vi "Get - SigMath Data.vi"(0 "reference in":refnum<class "SigMath.lvclass">, 5 "error in (no error)":errorcluster) -> (13 "SigMath Data":T1, 14 "reference out":refnum<class "SigMath.lvclass">, 19 "error out":errorcluster)   [LabVIEW 2020, in "SigMath.lvclass"]
uses:
  SigMath.lvclass
  protected/SigMath Data.ctl
  API/GSwFormDSP_class/GSwFormDSP.lvclass
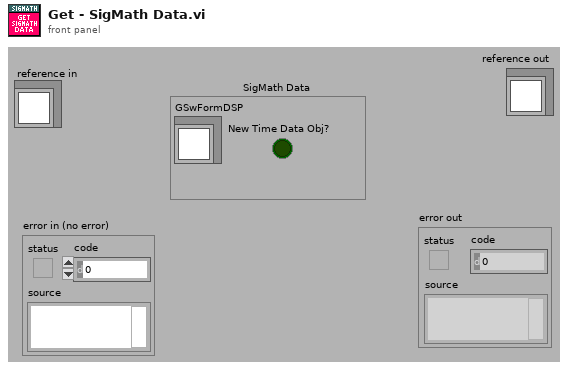
[diagram p1: front panel]
types:
  T1 = typedef "SigMath.lvclass/SigMath Data.ctl" = cluster{"New Time Data Obj?":bool, "GSwFormDSP":refnum<class "GSwFormDSP.lvclass">}
  T2 = typedef "SigMath.lvclass/ObjectAttributes.ctl" = cluster{"SigMath Data":T1, "User CTRL Refs":T3}
  T3 = typedef "SigMath.lvclass/SigMath User CTRL Refs.ctl" = cluster{"wForms":refnum<vi>, "Results wForms":refnum<vi>}
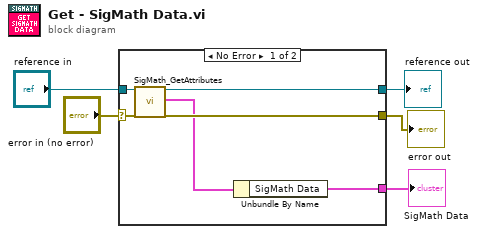
[diagram p0: block diagram]
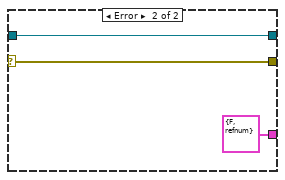
[diagram p2: hidden frame]
diagram:
  n1 = case shown="No Error" "error in (no error)" {
    selector: "error in (no error)" -> [w11 w14]
    tunnel: [w10 w14] -> w4
    tunnel: [w9 w13] -> w2
    tunnel: "reference in" -> [w7 w13]
    tunnel: [w6 T1 {"New Time Data Obj?"=FALSE, "GSwFormDSP"=refnum} ("BF Data")] -> w1
    frame No Error {
      n2 = call "SigMath_GetAttributes.vi"("reference in"=w7, "error in (no error)"=w11) -> ("reference out"=w9:refnum<class "SigMath.lvclass">, "attributes"=w8:T2, "error out"=w10:errorcluster)  [unwired: 14 in, 1 out]
      n3 = Unbundle By Name(w8) -> ("SigMath Data"=w6:T1)
    }
    frame Error {
    }
  }
  "error out" <- w4
  "reference out" <- w2
  "SigMath Data" <- w1
